vi "CalVal-Find Test Frequencies.vi"(9 "Unsmoothed":dbl[](array[numeric]), 10 "Smoothed":dbl[](array[numeric]), 11 "Frequency":dbl[](array[numeric])) -> (1 "Mags":dbl[](array[numeric]), 3 "Test Freqs":dbl[](array[numeric]))   [LabVIEW 2020]
uses:
  epl-vi-lib/Utility VIs/Array Manipulation VIs/Irregular Array Subset (DBL, Index).vi
  <vilib>/Analysis/NI_AAL_SigProc.lvlib
panel:
  out "Mag Graph":T1(graph)
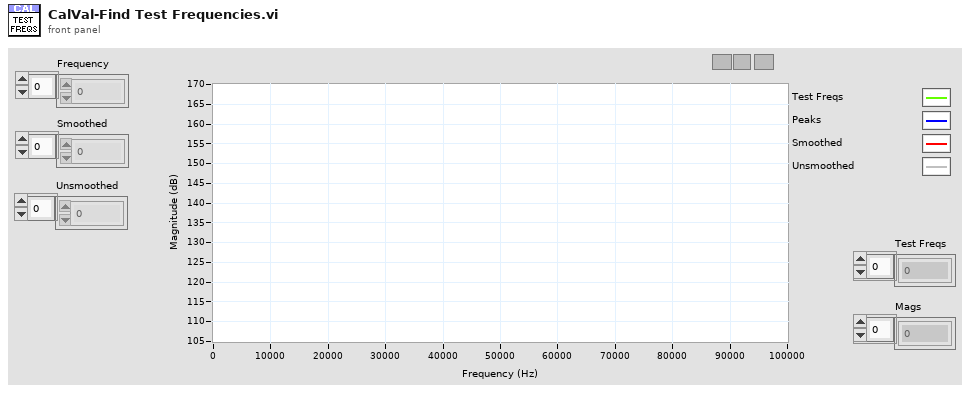
[diagram p1: front panel]
types:
  T1 = cluster{"Frequency (Hz)":dbl[], "Unsmoothed Mag":dbl[]}[]
  T2 = cluster{"Array Subset":dbl[], "Array Subset":dbl[]}
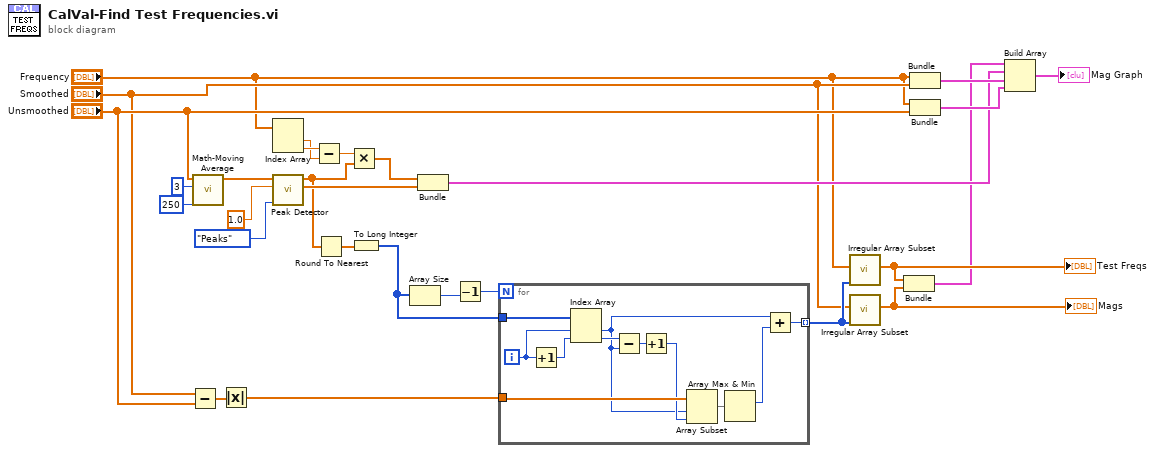
[diagram p0: block diagram]
diagram:
  n1 = Subtract(x="Smoothed", y="Unsmoothed") -> (x-y=w8:dbl[])
  n2 = call "Math-Moving Average.vi"("Iterations"=250, "Length"=3, "Array in"="Unsmoothed") -> ("Array out"=w18:dbl[])  [unwired: 8 in]
  n3 = Absolute Value(x=w8) -> (abs(x)=w7:dbl[])
  n4 = Index Array(array="Frequency") -> (element #1=w15:dbl, element #2=w16:dbl)  [unwired: 2 in]
  n5 = call <vilib>:"Peak Detector.vi"("peaks/valleys"=enum32{"Peaks", "Valleys"}."Peaks", "threshold"=1.0, "X"=w18) -> ("Amplitudes"=w23:dbl[], "Locations"=w13:dbl[])  [unwired: 4 in, 3 out]
  n6 = Subtract(x=w16, y=w15) -> (x-y=w14:dbl)
  n7 = Round To Nearest(number=w13) -> (nearest integer value=w24:dbl[])
  n8 = Multiply(x=w14, y=w13) -> (x*y=w21:dbl[])
  n9 = To Long Integer(number=w24) -> (32bit integer=w10:i32[])
  n10 = Array Size(array=w10) -> (size(s)=w12:i32)
  n11 = Bundle(w21, "Amplitudes"=w23) -> (w17:cluster{dbl[], "Amplitudes":dbl[]})  [unwired: 1 in]
  n12 = Decrement(x=w12) -> (x-1=w11:i32)
  n13 = for {
    N: w11 -> [_]
    tunnel: w10 -> [w39]
    tunnel: w7 -> [w36]
    tunnel: [w29] -> w6 mode=indexing
    i -> [w38]
    n14 = Increment(x=w38) -> (x+1=w37:i32)
    n15 = Index Array(array=w39, index #1=w38, index #2=w37) -> (element #1=w31:i32, element #2=w35:i32)
    n16 = Subtract(x=w35, y=w31) -> (x-y=w34:i32)
    n17 = Increment(x=w34) -> (x+1=w33:i32)
    n18 = Array Subset(array=w36, index=w31, length=w33) -> (w32:dbl[])
    n19 = Array Max & Min(array=w32) -> (max index (indices)=w30:i32)  [unwired: 3 out]
    n20 = Add(x=w31, y=w30) -> (x+y=w29:i32)
  }
  n21 = call-poly "Irregular Array Subset.vi"("Indices"=w6, "Array"="Frequency") -> ("Array Subset"=w3:dbl[])  [unwired: 8 in, 1 out]
  "Test Freqs" <- w3
  n22 = call-poly "Irregular Array Subset.vi"("Indices"=w6, "Array"="Smoothed") -> ("Array Subset"=w2:dbl[])  [unwired: 8 in, 1 out]
  "Mags" <- w2
  n23 = Bundle("Array Subset"=w3, "Array Subset"=w2) -> (w1:T2)  [unwired: 1 in]
  n24 = Bundle("Frequency"="Frequency", "Smoothed"="Smoothed") -> (w28:cluster{"Frequency":dbl[], "Smoothed":dbl[]})  [unwired: 1 in]
  n25 = Bundle("Frequency"="Frequency", "Unsmoothed"="Unsmoothed") -> (w27:cluster{"Frequency":dbl[], "Unsmoothed":dbl[]})  [unwired: 1 in]
  n26 = Build Array(w1, w17, w28, w27) -> (→"Mag Graph":cluster{"Frequency":dbl[], "Unsmoothed":dbl[]}[])
